vi "VentCheck.vi"(8 "error in (no error)":errorcluster, 11 "UI.lvclass":refnum<class "S1.lvclass">) -> (0 "error out":errorcluster)   [LabVIEW 2018, in "S1.lvclass"]
uses:
  S1.lvclass
  S1.lvclass/S1.ctl
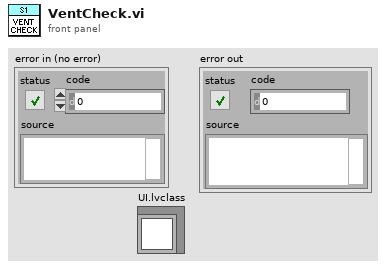
[diagram p1: front panel]
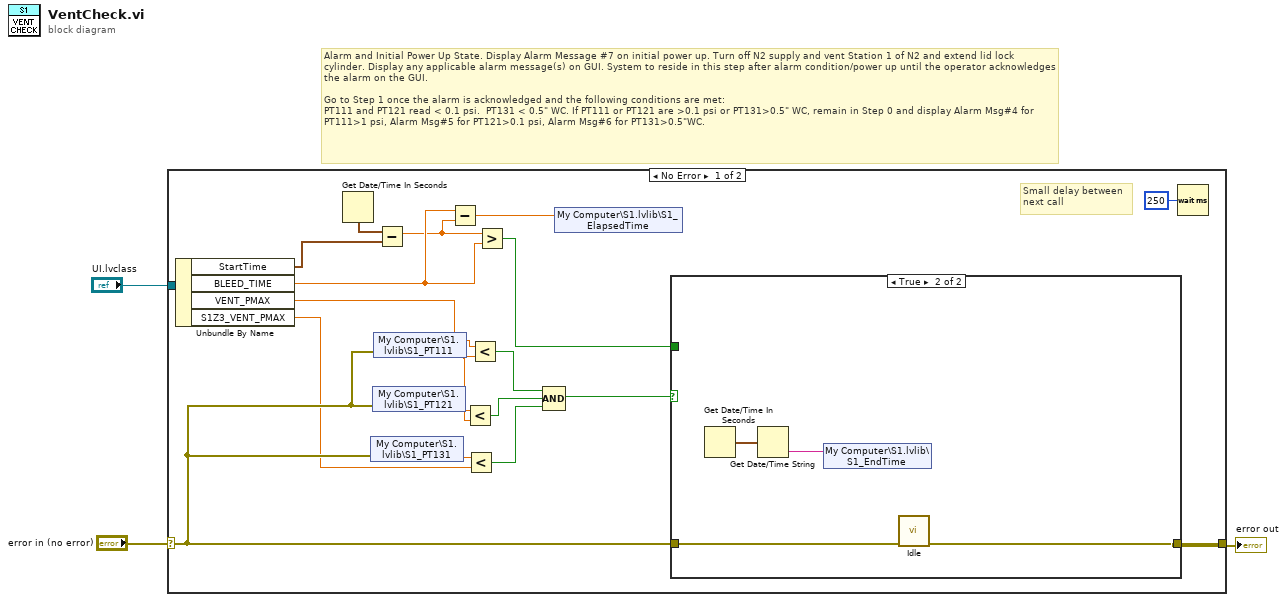
[diagram p0: block diagram]
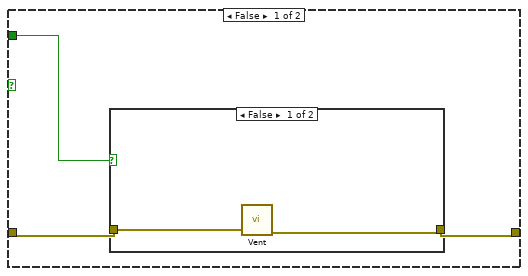
[diagram p2: hidden frame]
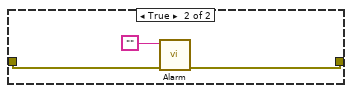
[diagram p3: hidden frame]
diagram:
  # "Alarm and Initial Power Up State. Display Alarm Message #7 on initial power up. Turn off N2 supply and vent Station 1 of N2 and extend lid lock cylinder. Display any applicable alarm message(s) on GUI. System to reside in this step after alarm condition/power up until the operator acknowledges the alarm on the GUI. \n\nGo to Step 1 once the alarm is acknowledged and the following conditions are met:\nPT111 and PT121 read < 0.1 psi.  PT131 < 0.5\" WC. If PT111 or PT121 are >0.1 psi or PT131>0.5\" WC, remain in Step 0 and display Alarm Msg#4 for PT111>1 psi, Alarm Msg#5 for PT121>0.1 psi, Alarm Msg#6 for PT131>0.5\"WC."
  n1 = case shown="No Error" "error in (no error)" {
    selector: "error in (no error)" -> [w14 w35]
    tunnel: [w18 w35] -> w2
    tunnel: "UI.lvclass" -> [w10 _]
    frame No Error {
      # "Small delay between\nnext call"
      n2 = Unbundle By Name(w10) -> ("StartTime"=w4:timestamp, "BLEED_TIME"=w9:dbl, "VENT_PMAX"=w6:dbl, "S1Z3_VENT_PMAX"=w5:dbl)
      n3 = Get Date/Time In Seconds() -> (seconds since 1Jan1904=w12:timestamp)
      n4 = shared-variable "My Computer\\S1.lvlib\\S1_PT131"(error in=w14) -> (w20:dbl)  [unwired: 1 out]
      n5 = shared-variable "My Computer\\S1.lvlib\\S1_PT121"(error in=w14) -> (w21:dbl)  [unwired: 1 out]
      n6 = shared-variable "My Computer\\S1.lvlib\\S1_PT111"(error in=w14) -> (w22:dbl)  [unwired: 1 out]
      n7 = Subtract(x=w12, y=w4) -> (x-y=w8:dbl)
      n8 = Subtract(x=w9, y=w8) -> (x-y=w7:dbl)
      n9 = Less?(x=w21, y=w6) -> (x < y?=w16:bool)
      n10 = Less?(x=w20, y=w5) -> (x < y?=w15:bool)
      n11 = Less?(x=w22, y=w6) -> (x < y?=w17:bool)
      n12 = Greater?(x=w8, y=w9) -> (0:w11:bool)
      n13 = Compound Arithmetic op=AND(w17, w16, w15) -> (w19:bool)
      n14 = shared-variable "My Computer\\S1.lvlib\\S1_ElapsedTime"(w7) -> ()  [unwired: 1 in, 1 out]
      n15 = case shown="True" w19 {
        tunnel: w14 -> [w24 w34]
        tunnel: [w25 w33] -> w18
        tunnel: w11 -> [w23 _]
        frame False {
          n16 = case shown="False" w23 {
            tunnel: [w26 w30] -> w25
            tunnel: w24 -> [w27 w29]
            frame False {
              n17 = call "Vent.vi"("error in"=w27) -> ("error out"=w26:errorcluster)  [unwired: 10 in]
            }
            frame True {
              n18 = call "Alarm.vi"("error in"=w29, "Alarm"="") -> ("error out"=w30:errorcluster)  [unwired: 9 in]
            }
          }
        }
        frame True {
          n19 = Get Date/Time In Seconds() -> (seconds since 1Jan1904=w32:timestamp)
          n20 = Get Date/Time String(seconds (now)=w32) -> (time string=w31:string)  [unwired: 2 in, 1 out]
          n21 = shared-variable "My Computer\\S1.lvlib\\S1_EndTime"(w31) -> ()  [unwired: 1 in, 1 out]
          n22 = call "Idle.vi"("error in"=w34) -> ("error out"=w33:errorcluster)  [unwired: 10 in]
        }
      }
      n23 = Wait (ms)(milliseconds to wait=u32 250) -> ()  [unwired: 1 out]
    }
    frame Error {
    }
  }
  "error out" <- w2
